vi "Check For Amps on v1.vi"(10 "ID":string, 11 "amps":dbl) -> (3 "amps":bool)   [LabVIEW 2017]
uses:
  program files/Global display 3.vi
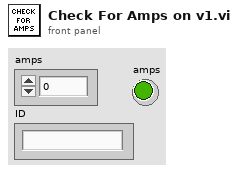
[diagram p1: front panel]
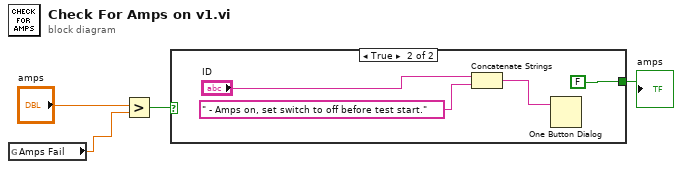
[diagram p0: block diagram]
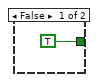
[diagram p2: hidden frame]
diagram:
  n1 = global read "Global display 3.vi" "Amps Fail"() -> (w1:dbl)
  n2 = Greater?(x="amps", y=w1) -> (0:w3:bool)
  n3 = case shown="True" w3 {
    tunnel: [TRUE FALSE] -> w2
    frame False {
    }
    frame True {
      n4 = Concatenate Strings("ID", " - Amps on, set switch to off before test start.") -> (w6:string)
      n5 = One Button Dialog(message=w6) -> ()  [unwired: 1 in, 1 out]
    }
  }
  "amps" <- w2
